vi "2.vi"() -> ()   [LabVIEW 2014]
panel:
  in  "Array Sixe":dbl
  out "Array":dbl[](array[numeric])
  in  "Max RNG":dbl
  in  "Min RNG":dbl
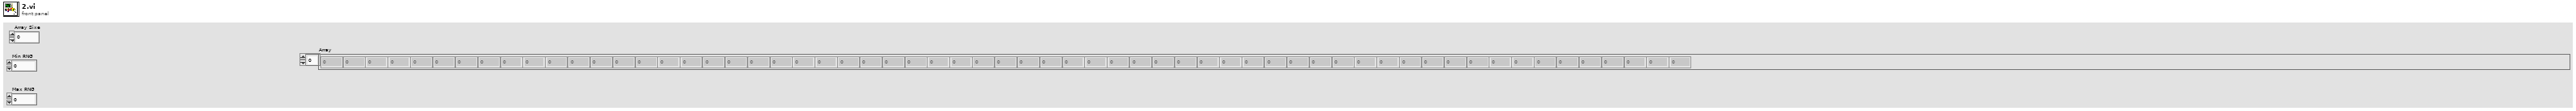
[diagram p1: front panel]
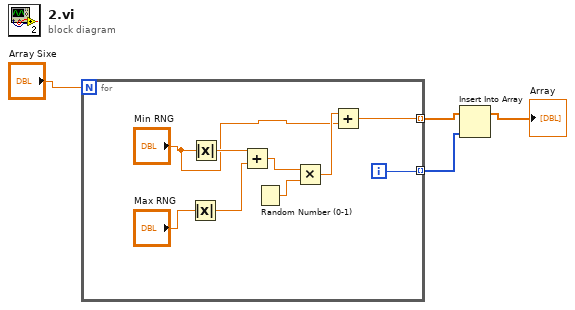
[diagram p0: block diagram]
diagram:
  n1 = for {
    N: "Array Sixe" -> [_]
    tunnel: [w6] -> w2 mode=indexing
    tunnel: [w5] -> w1 mode=indexing
    i -> [w5]
    n2 = Absolute Value(x="Max RNG") -> (abs(x)=w12:dbl)
    n3 = Absolute Value(x="Min RNG") -> (abs(x)=w8:dbl)
    n4 = Add(x=w8, y=w12) -> (x+y=w11:dbl)
    n5 = Random Number (0-1)() -> (number: 0 to 1=w10:dbl)
    n6 = Multiply(x=w11, y=w10) -> (x*y=w9:dbl)
    n7 = Add(x=w9, y="Min RNG") -> (x+y=w6:dbl)
  }
  n8 = Insert Into Array(array=w2, new element=w1) -> (→"Array":dbl[])  [unwired: 1 in]
